vi "APDM Allocate New Context.vi"(2 "error in (no error)":errorcluster, 3 "APDM Context In":T1={"APDM Context ID"=0, "Gyro Mode"="", "Log Data"=FALSE, "Log File"=refnum, "Gyro Record Log"=refnum, "Gyro CMD Log"=refnum, "L Opal SN"=0, "R Opal SN"=0, "Access Point ID"=0, "Left Gyro Sim Data"=path "C:/Users/jfalesi/Desktop/CP FES Walking Code/Original/Ahad Vi/CP Code/Offline data/TD_7_Raw_R.txt", "Right Gyro Sim Data"=path "C:/Users/jfalesi/Desktop/CP FES Walking Code/Original/Ahad Vi/CP Code/Offline data/TD_7_Raw_R.txt", "Sampling Rate"=0.0, "Gyro Sim Time Array"=[], "Missed Gyro Count"=0.0}) -> (0 "error out":errorcluster, 1 "APDM Context Out":T1={"APDM Context ID"=0, "Gyro Mode"="", "Log Data"=FALSE, "Log File"=refnum, "Gyro Record Log"=refnum, "Gyro CMD Log"=refnum, "L Opal SN"=0, "R Opal SN"=0, "Access Point ID"=0, "Left Gyro Sim Data"=path "C:/Users/jfalesi/Desktop/CP FES Walking Code/Original/Ahad Vi/CP Code/Offline data/TD_7_Raw_R.txt", "Right Gyro Sim Data"=path "C:/Users/jfalesi/Desktop/CP FES Walking Code/Original/Ahad Vi/CP Code/Offline data/TD_7_Raw_R.txt", "Sampling Rate"=0.0, "Gyro Sim Time Array"=[], "Missed Gyro Count"=0.0})   [LabVIEW 2019]
uses:
  Controls/APDM Context Cluster.ctl
  Lee Lab/CP FES Walking 2018/Code/Working/LabVIEW/apdm.dll
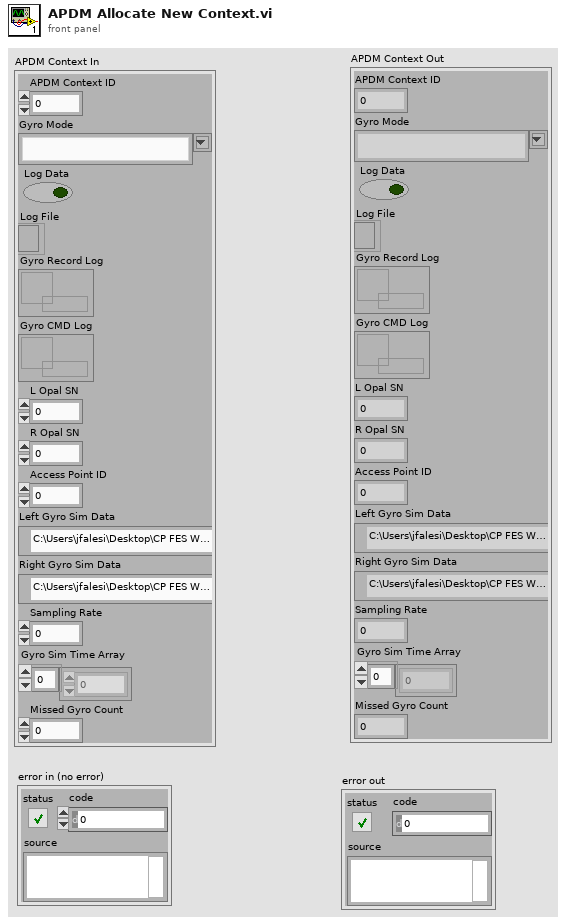
[diagram p1: front panel]
types:
  T1 = typedef "APDM Context Cluster.ctl" = cluster{"APDM Context ID":u32, "Gyro Mode":string, "Log Data":bool, "Log File":refnum<file>, "Gyro Record Log":refnum<queue>, "Gyro CMD Log":refnum<queue>, "L Opal SN":u32, "R Opal SN":u32, "Access Point ID":u32, "Left Gyro Sim Data":path, "Right Gyro Sim Data":path, "Sampling Rate":dbl, "Gyro Sim Time Array":dbl[], "Missed Gyro Count":dbl}
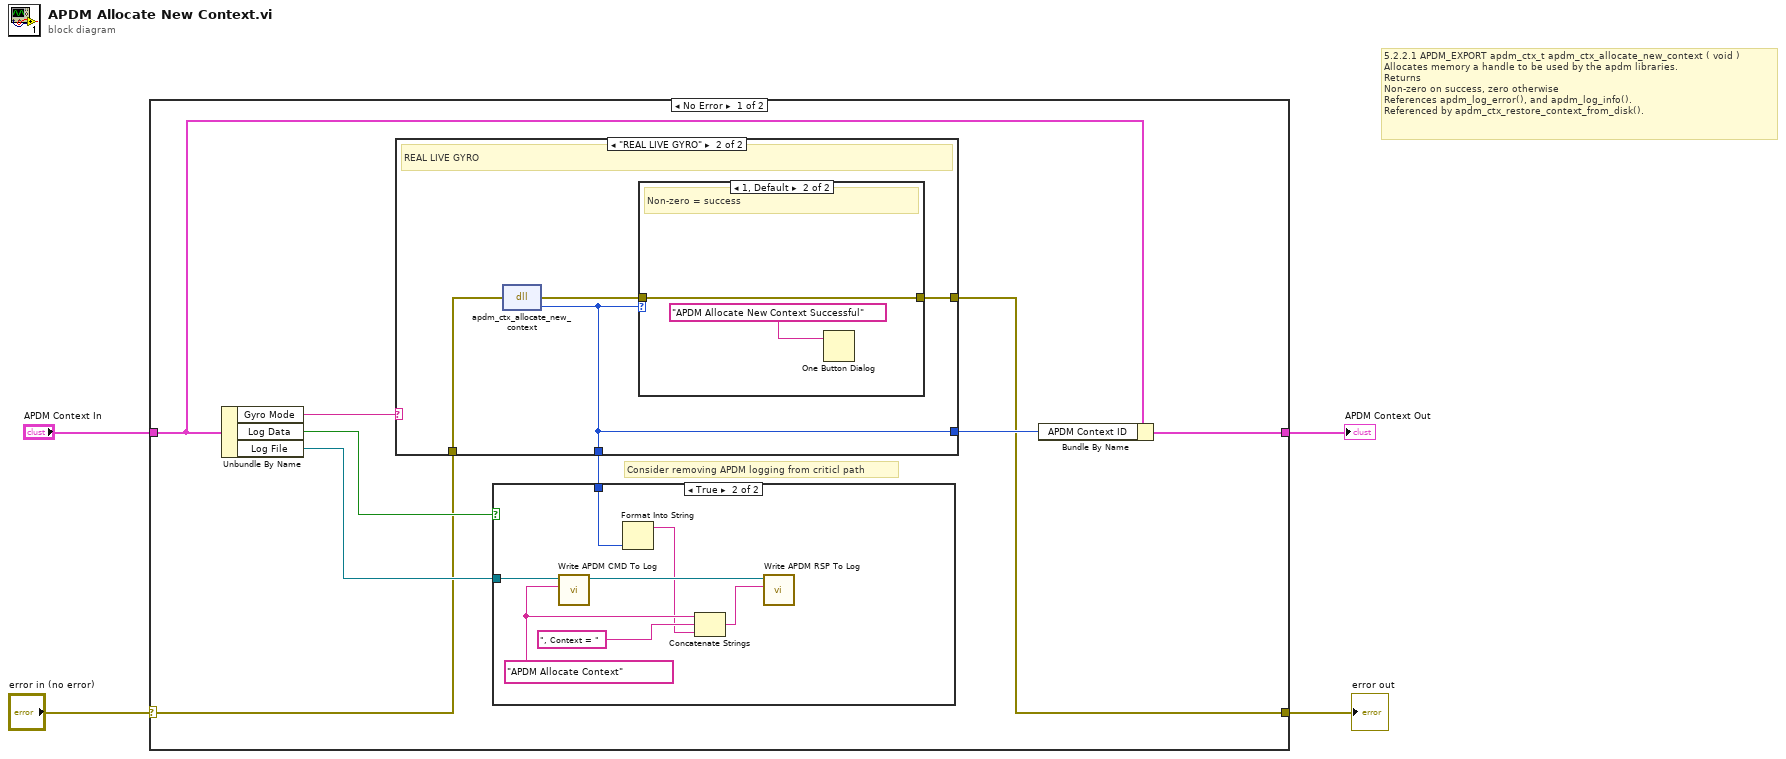
[diagram p0: block diagram]
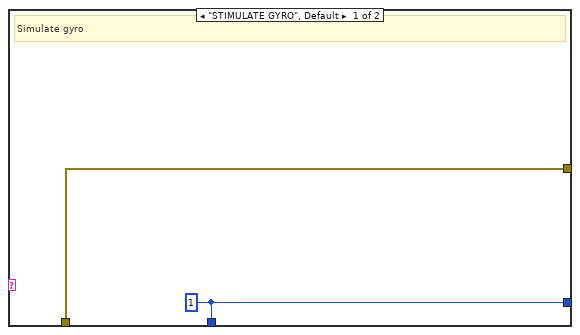
[diagram p3: hidden frame]
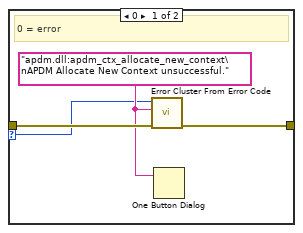
[diagram p4: hidden frame]
diagram:
  # "5.2.2.1 APDM_EXPORT apdm_ctx_t apdm_ctx_allocate_new_context ( void )\nAllocates memory a handle to be used by the apdm libraries.\nReturns\nNon-zero on success, zero otherwise\nReferences apdm_log_error(), and apdm_log_info().\nReferenced by apdm_ctx_restore_context_from_disk()."
  n1 = case shown="No Error" "error in (no error)" {
    selector: "error in (no error)" -> [w8 w34]
    tunnel: [w7 w34] -> w3
    tunnel: "APDM Context In" -> [w6 w33]
    tunnel: [w5 w33] -> w1
    frame No Error {
      # "Consider removing APDM logging from criticl path"
      n2 = Unbundle By Name(w6) -> ("Gyro Mode"=w12:string, "Log Data"=w11:bool, "Log File"=w10:refnum<file>)
      n3 = case shown="\"REAL LIVE GYRO\"" w12 {
        tunnel: [w22 w24] -> w9
        tunnel: [w22 w24] -> w13
        tunnel: [w21 w23] -> w7
        tunnel: w8 -> [w21 w26]
        frame "STIMULATE GYRO", Default {
          w22 = 1
          # "Simulate gyro"
        }
        frame "REAL LIVE GYRO" {
          # "REAL LIVE GYRO"
          n4 = dll-call lib="C:/Users/jfalesi/Dropbox/Lee Lab/CP FES Walking 2018/Code/Working/LabVIEW/apdm.dll" fn="apdm_ctx_allocate_new_context"(error in=w26) -> (error out=w25:errorcluster, "return type"=w24:u32)  [unwired: 2 in, 1 out]
          n5 = case shown="1, Default" w24 {
            selector: w24 -> [w27 _]
            tunnel: w25 -> [w30 w32]
            tunnel: [w29 w32] -> w23
            frame 0 {
              w28 = "apdm.dll:apdm_ctx_allocate_new_context\nAPDM Allocate New Context unsuccessful." ("message")
              # "0 = error"
              n6 = call <vilib>:"Error Cluster From Error Code.vi"("error in (no error)"=w30, "error message (\"\")"=w28, "error code (0)"=w27) -> ("error out"=w29:errorcluster)  [unwired: 6 in]
              n7 = One Button Dialog(message=w28) -> ()  [unwired: 1 in, 1 out]
            }
            frame 1, Default {
              # "Non-zero = success"
              n8 = One Button Dialog(message="APDM Allocate New Context Successful") -> ()  [unwired: 1 in, 1 out]
            }
          }
        }
      }
      n9 = case shown="True" w11 {
        tunnel: w13 -> [_ w19]
        tunnel: w10 -> [_ w14]
        frame False {
        }
        frame True {
          w17 = "APDM Allocate Context" ("Log Item")
          n10 = call "Write APDM CMD To Log.vi"("Log Item"=w17, "Byte Stream File in"=w14) -> ("Byte Stream File out"=w20:refnum<file>)  [unwired: 8 in, 1 out]
          n11 = Format Into String "Format Into String"(w19) -> (resulting string=w15:string)  [unwired: 3 in, 1 out]
          n12 = Concatenate Strings(w17, ", Context = " ("string"), w15) -> (w18:string)
          n13 = call "Write APDM RSP To Log.vi"("Log Item"=w18, "Byte Stream File in"=w20) -> ()  [unwired: 9 in, 1 out]
        }
      }
      n14 = Bundle By Name(cluster=w6, "APDM Context ID"=w9) -> (w5:T1)
    }
    frame Error {
    }
  }
  "error out" <- w3
  "APDM Context Out" <- w1
